vi "Delta acquire.vi"(8 "error in (no error)":errorcluster, 11 "VISA Resource In":refnum<visa-resource-name>) -> (0 "error out":errorcluster, 3 "Resource Out":refnum<visa-resource-name>, 4 "Y Value":dbl, 5 "X Value":dbl)   [LabVIEW 2023]
uses:
  <instrlib>/Keithley 622x LV 2009/Utility/Status Registers/Typedefs/KE622x -- Meas Event Reg State.ctl
  <instrlib>/Keithley 622x LV 2009/Action-Status/Typedefs/KE622x -- Math Result Type.ctl
  <instrlib>/Keithley 622x LV 2009/Keithley 622x.lvlib
panel:
  out "KE622x Meas Event Reg":T1
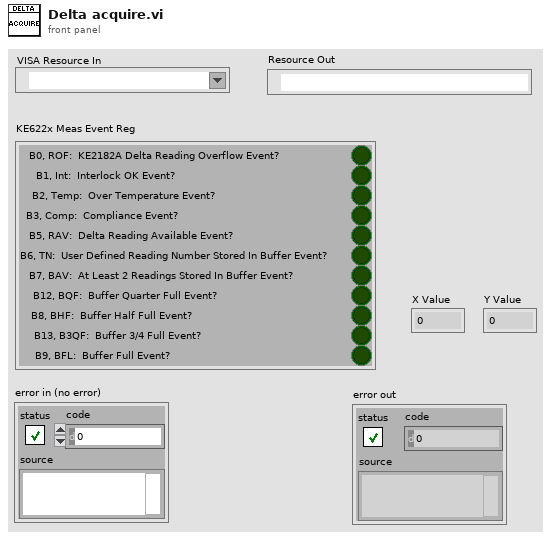
[diagram p1: front panel]
types:
  T1 = typedef "Keithley 622x.lvlib/KE622x -- Meas Event Reg State.ctl" = cluster{"B0, ROF:  KE2182A Delta Reading Overflow Event?":bool, "B1, Int:  Interlock OK Event?":bool, "B2, Temp:  Over Temperature Event?":bool, "B3, Comp:  Compliance Event?":bool, "B5, RAV:  Delta Reading Available Event?":bool, "B6, TN:  User Defined Reading Number Stored In Buffer Event?":bool, "B7, BAV:  At Least 2 Readings Stored In Buffer Event?":bool, "B12, BQF:  Buffer Quarter Full Event?":bool, "B8, BHF:  Buffer Half Full Event?":bool, "B13, B3QF:  Buffer 3/4 Full Event?":bool, "B9, BFL:  Buffer Full Event?":bool}
  T2 = typedef "Keithley 622x.lvlib/KE622x -- Math Result Type.ctl" = enum16{"Latest", "Fresh"}
  T3 = typedef "Keithley 622x.lvlib/KE622x -- Math Results.ctl" = cluster{"X Value":dbl, "Y Value":dbl}
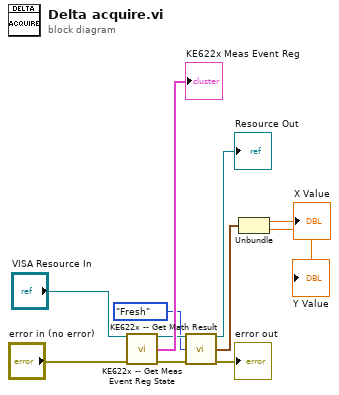
[diagram p0: block diagram]
diagram:
  n1 = call <instrlib>:"KE622x -- Get Meas Event Reg State.vi"("VISA Resource In"="VISA Resource In", "error in (no error)"="error in (no error)") -> ("VISA Resource Out (dupl)"=w8:refnum<visa-resource-name>, "KE622x Meas Event Reg"=→"KE622x Meas Event Reg":T1, "error out"=w9:errorcluster)  [unwired: 11 in]
  n2 = call <instrlib>:"KE622x -- Get Math Result.vi"("Resource In"=w8, "Result Type"=KE622x_--_Math_Result_Type."Fresh", "error in (no error)"=w9) -> ("Resource Out (dupl)"=→"Resource Out":refnum<visa-resource-name>, "Math Results"=w11:T3, "error out"=→"error out":errorcluster)  [unwired: 10 in]
  n3 = Unbundle(w11) -> ("X Value"=→"X Value":dbl, "Y Value"=→"Y Value":dbl)
